vi "反算.vi"(8 "error in (no error)":errorcluster caption="错误输入（无错误）", 10 "公式":cluster{"X^2":dbl, "X":dbl, "B":dbl}, 11 "监测值":dbl) -> (0 "error out":errorcluster caption="错误输出", 3 "信号值":dbl)   [LabVIEW 2016, in "random number.lvlib"]
uses:
  random number.lvlib
  <vilib>/Analysis/polynomials.llb/Polynomial Roots (DBL).vi
  <vilib>/Analysis/polynomials.llb/Polynomial Plot (Range).vi
  <vilib>/Analysis/NI_AALPro.lvlib
panel:
  out "Real Roots":dbl[](array[numeric]) caption="实数根"
  out "polynomial plot":cluster{dbl[], "P(A)":dbl[]}(graph) caption="多项式曲线"
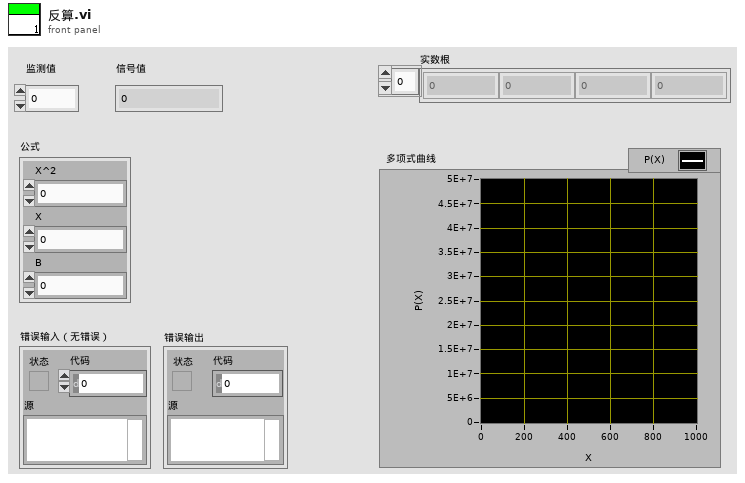
[diagram p1: front panel]
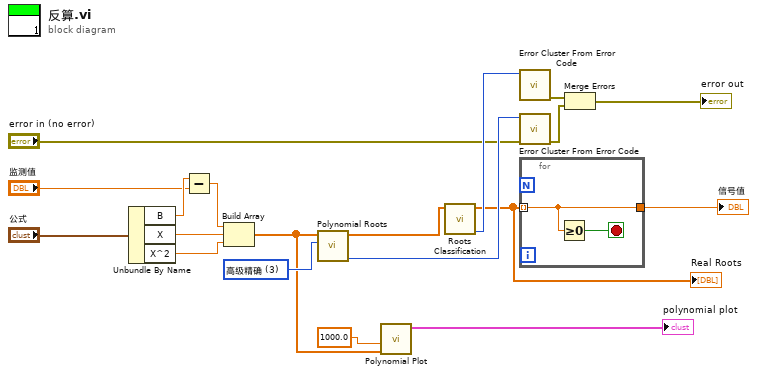
[diagram p0: block diagram]
diagram:
  w19 = u16 3 items=["常规", "简单分类", "精确", "高级精确"] ("option")
  n1 = Unbundle By Name("公式") -> ("B"=w17:dbl, "X"=w14:dbl, "X^2"=w13:dbl)
  n2 = Subtract(x=w17, y="监测值") -> (x-y=w15:dbl)
  n3 = Build Array(w15, w14, w13) -> (w11:dbl[])
  n4 = call-poly <vilib>:"Polynomial Roots.vi"("option"=w19, "P(x)"=w11) -> ("error"=w12:i32, "Roots"=w9:cdb[])  [unwired: 8 in]
  n5 = call-poly <vilib>:"Polynomial Plot.vi"("P(x)"=w11, "end"=1000.0) -> ("polynomial plot"=→"polynomial plot":cluster{"Ramp Pattern":dbl[], "P(A)":dbl[]})  [unwired: 8 in, 1 out]
  n6 = call <vilib>:"Roots Classification.vi"("Roots"=w9) -> ("error"=w7:i32, "Real Roots"=w3:dbl[])  [unwired: 7 in, 2 out]
  "Real Roots" <- w3
  n7 = call <vilib>:"Error Cluster From Error Code.vi"("error code (0)"=w7) -> ("error out"=w6:errorcluster)  [unwired: 8 in]
  n8 = call <vilib>:"Error Cluster From Error Code.vi"("error in (no error)"="error in (no error)", "error code (0)"=w12) -> ("error out"=w5:errorcluster)  [unwired: 7 in]
  n9 = for {
    tunnel: w3 -> [w21] mode=indexing
    tunnel: [w21] -> w2
    stop <- w20 stop-if-true
    n10 = Greater Or Equal To 0?(x=w21) -> (x >= 0?=w20:bool)
  }
  "信号值" <- w2
  n11 = Merge Errors(w6, w5) -> (→"error out":errorcluster)
